vi "Set ChildNode subpanel.vi"(8 "error in (no error)":errorcluster caption="错误输入（无错误）", 11 "ParentDataNode in":refnum<class "PanelDataNode.lvclass"> caption="DNL_LabVIEW Object in") -> (0 "error out":errorcluster caption="错误输出", 2 "ChildDataNode[]":refnum<data-value>[](array[refnum]), 3 "ParentDataNode out":refnum<class "PanelDataNode.lvclass"> caption="DNL_LabVIEW Object out")   [LabVIEW 2013, in "PanelDataNode.lvclass"]
uses:
  PanelDataNode.lvclass
  PanelLinkNode/PanelLinkNode.lvclass/PanelLinkNode.ctl
  PanelDataNode.lvclass/PanelDataNode.ctl
  PanelLinkNode/PanelLinkNode.lvclass
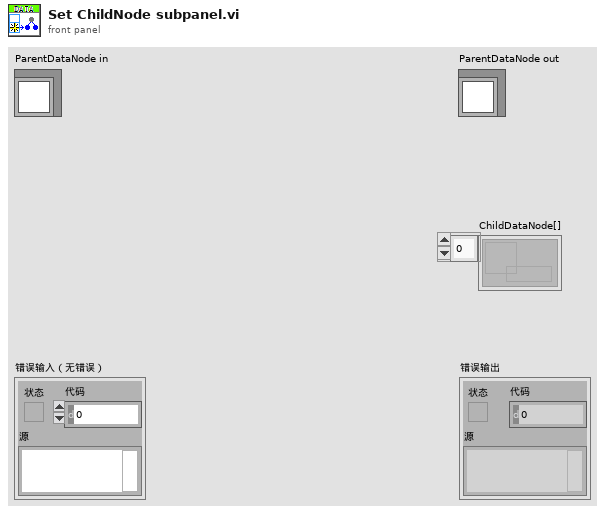
[diagram p1: front panel]
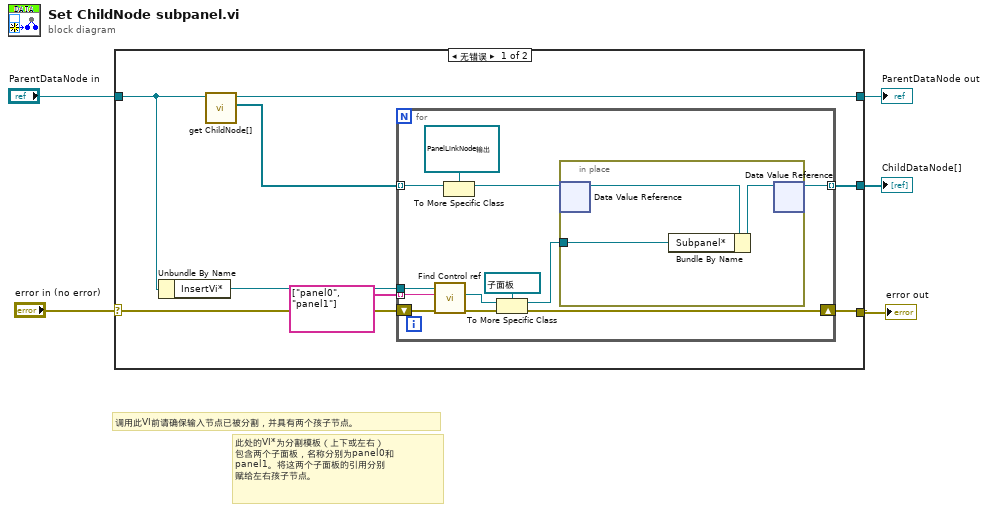
[diagram p0: block diagram]
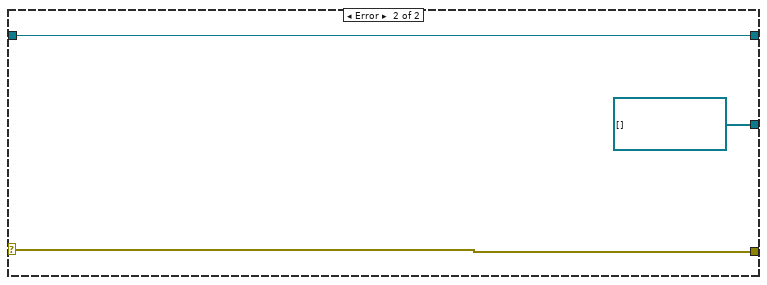
[diagram p2: hidden frame]
diagram:
  # "此处的VI*为分割模板（上下或左右）\n包含两个子面板，名称分别为panel0和\npanel1。将这两个子面板的引用分别\n赋给左右孩子节点。"
  # "调用此VI前请确保输入节点已被分割，并具有两个孩子节点。"
  n1 = case shown="无错误" "error in (no error)" {
    selector: "error in (no error)" -> [w12 w31]
    tunnel: [w10 w31] -> w4
    tunnel: [w9 w30] -> w2
    tunnel: "ParentDataNode in" -> [w11 w30]
    tunnel: [w6 refnum<data-value>[] []] -> w1
    frame No Error {
      n2 = Unbundle By Name(w11) -> ("InsertVi*"=w13:refnum<vi>)
      n3 = call "get ChildNode[].vi"("PanelLinkNode输入"=w11) -> ("ChildNode*[]"=w8:refnum<data-value>[], "PanelLinkNode输出"=w9:refnum<class "PanelDataNode.lvclass">)  [unwired: 8 in, 1 out]
      n4 = for {
        tunnel: string[] ["panel0", "panel1"] -> [w25] mode=indexing
        tunnel: w13 -> [w24]
        shift-right: [w14] -> w10
        shift-left: w12 -> [w18]
        tunnel: w8 -> [w17] mode=indexing
        tunnel: [w16] -> w6 mode=indexing
        n5 = call "Find Control ref.vi"("error in (no error)"=w18, "control name"=w25, "panelvi*"=w24) -> ("error out"=w15:errorcluster, "ctrl*"=w21:refnum<vi>)  [unwired: 6 in, 1 out]
        n6 = To More Specific Class(target class=refnum<data-value> refnum ("数据值引用"), reference=w17) -> (specific class reference=w23:refnum<data-value>)  [unwired: 1 in, 1 out]
        n7 = To More Specific Class(target class=refnum<vi> refnum ("Subpanel*"), reference=w21, error in=w15) -> (specific class reference=w20:refnum<vi>, error out=w14:errorcluster)
        n8 = in-place {
          in-place-border: w20 -> [w27]
          n9 = in-place-dvr #1(w23) -> (w28:refnum<class "PanelDataNode.lvclass">)  [unwired: 1 out]
          n10 = Bundle By Name(cluster=w28, "Subpanel*"=w27) -> (w26:refnum<class "PanelDataNode.lvclass">)
          n11 = in-place-dvr #1(w26) -> (w16:refnum<data-value>)  [unwired: 1 out]
        }
      }
    }
    frame Error {
    }
  }
  "error out" <- w4
  "ParentDataNode out" <- w2
  "ChildDataNode[]" <- w1
